vi "gestosc_widoma_en_mocy_SubVi.vi"(11 "signal in":waveform(dbl)) -> (2 "gestosc widmowa mocy":waveform(dbl)(graph), 3 "gestosc widmowa energii":waveform(dbl)(graph))   [LabVIEW 2025]
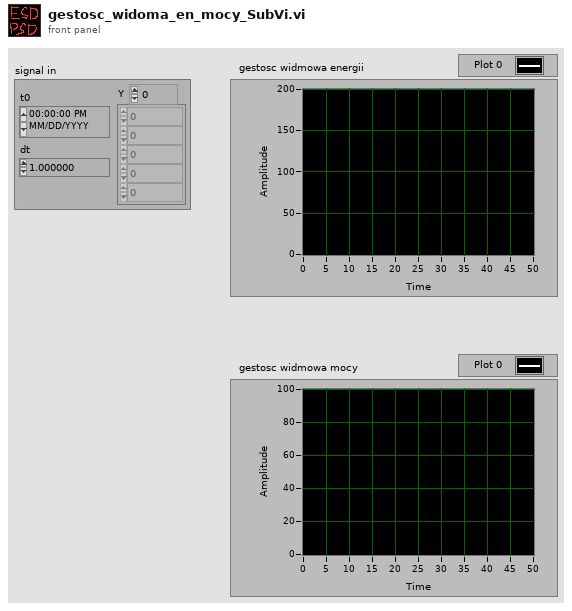
[diagram p1: front panel]
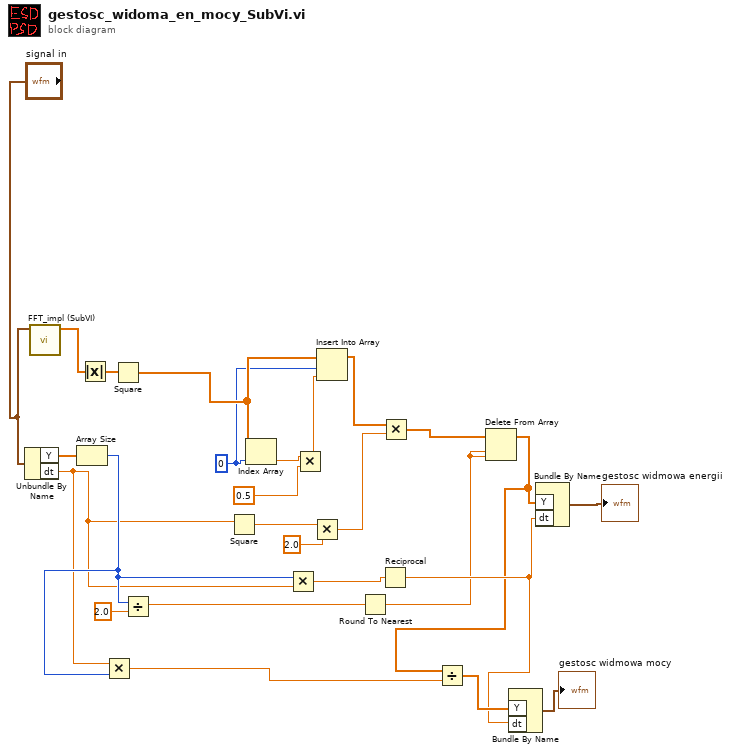
[diagram p0: block diagram]
diagram:
  w9 = 0 ("index")
  n1 = Unbundle By Name("signal in") -> ("Y"=w10:dbl[], "dt"=w20:dbl)
  n2 = call "FFT_impl (SubVI).vi"("Array"="signal in") -> ("FFT{x}"=w1:cdb[])  [unwired: 10 in]
  n3 = Array Size(array=w10) -> (size(s)=w21:i32)
  n4 = Absolute Value(x=w1) -> (abs(x)=w18:dbl[])
  n5 = Multiply(x=w20, y=w21) -> (x*y=w24:dbl)
  n6 = Square(x=w18) -> (x^2=w19:dbl[])
  n7 = Divide(x=w21, y=2.0) -> (x/y=w3:dbl)
  n8 = Square(x=w20) -> (x^2=w12:dbl)
  n9 = Index Array(array=w19, index=w9) -> (element=w8:dbl)
  n10 = Multiply(x=w21, y=w20) -> (x*y=w17:dbl)
  n11 = Multiply(x=w8, y=0.5 ("index")) -> (x*y=w6:dbl)
  n12 = Multiply(x=w12, y=2.0) -> (x*y=w16:dbl)
  n13 = Insert Into Array(array=w19, index=w9, new element=w6) -> (w14:dbl[])
  n14 = Round To Nearest(number=w3) -> (nearest integer value=w11:dbl)
  n15 = Reciprocal(x=w17) -> (1/x=w25:dbl)
  n16 = Multiply(x=w14, y=w16) -> (x*y=w15:dbl[])
  n17 = Delete From Array(array=w15, length=w11, index=w11) -> (array with subset deleted=w23:dbl[])  [unwired: 1 out]
  n18 = Divide(x=w23, y=w24) -> (x/y=w26:dbl[])
  n19 = Bundle By Name("Y"=w26, "dt"=w25) -> (→"gestosc widmowa mocy":waveform(dbl))  [unwired: 1 in]
  n20 = Bundle By Name("Y"=w23, "dt"=w25) -> (→"gestosc widmowa energii":waveform(dbl))  [unwired: 1 in]
